vi "test Cancelling an Already Cancelled Test Is A No Op.vi"(8 "error in (no error)":errorcluster, 11 "TestCase in":refnum<class "Cancellation Tests.lvclass">) -> (0 "error out":errorcluster, 3 "TestCase out":refnum<class "Cancellation Tests.lvclass">)   [LabVIEW 2017, in "Cancellation Tests.lvclass"]
uses:
  Cancellation Tests.lvclass
  <vilib>/addons/_JKI Toolkits/VI Tester/TestCase.llb/TestCase.lvclass
  Futures/Futures.lvlib
  Futures/Future/Future.lvclass
  C:/Program Files (x86)/National Instruments/LabVIEW 2017/vi.lib/addons/_JKI Toolkits/VI Tester/TestCase.llb/TestCase.lvclass
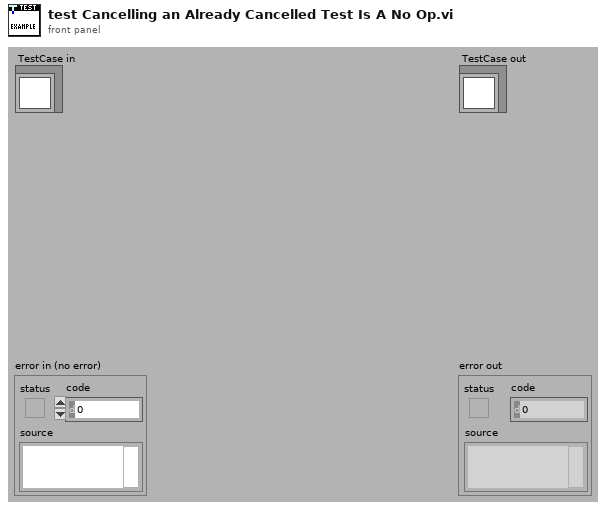
[diagram p1: front panel]
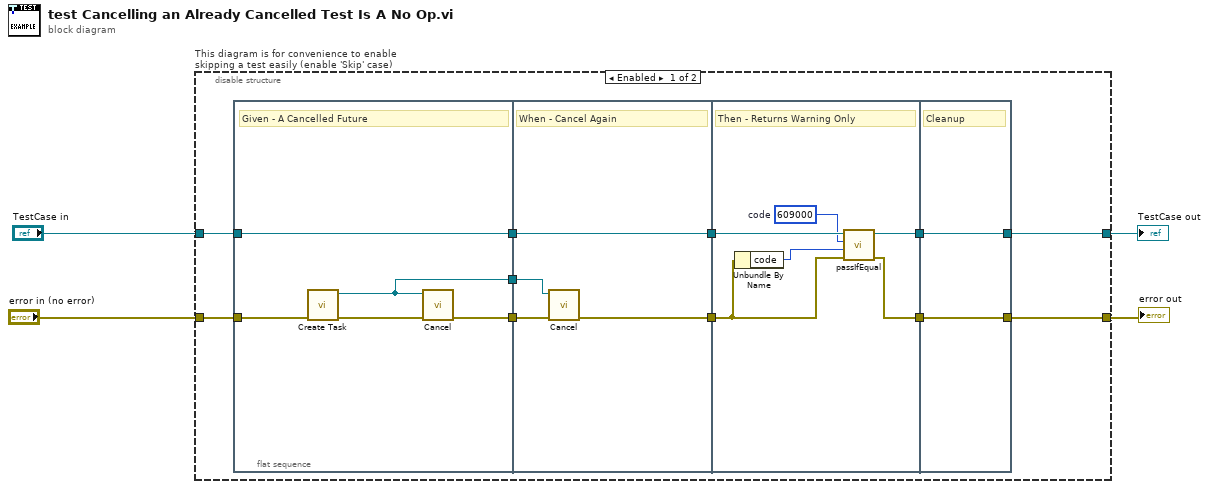
[diagram p0: block diagram]
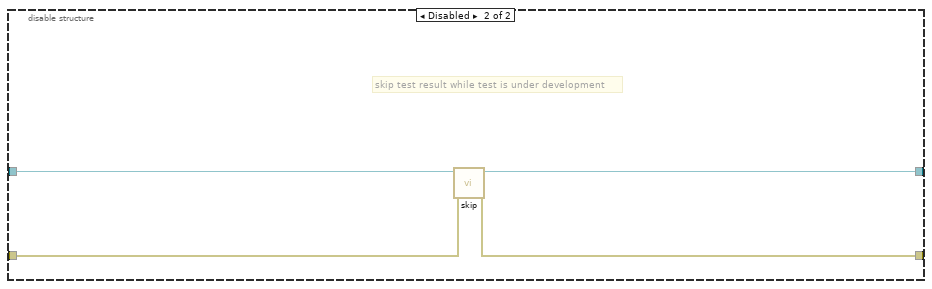
[diagram p2: hidden frame]
diagram:
  n1 = disable-structure "This diagram is for convenience to enable skipping a test easily (enable 'Skip' case)" shown="Enabled" {
    disable-tunnel: "TestCase in" -> [w11 w36]
    disable-tunnel: [w9 w34] -> w1
    disable-tunnel: [w8 w35] -> w3
    disable-tunnel: "error in (no error)" -> [w10 w33]
    frame Enabled {
      n2 = flat-sequence {
        tunnel: w10 -> [w19]
        tunnel: w11 -> [w20]
        tunnel: [w20] -> w15
        tunnel: [w17] -> w7
        tunnel: [w16] -> w6
        tunnel: [w24] -> w14
        tunnel: w15 -> [w24]
        tunnel: w7 -> [w23]
        tunnel: w6 -> [w22]
        tunnel: [w21] -> w5
        tunnel: [w28] -> w13
        tunnel: [w30] -> w12
        tunnel: w14 -> [w29]
        tunnel: w5 -> [w27]
        tunnel: [w31] -> w8
        tunnel: [w32] -> w9
        tunnel: w13 -> [w32]
        tunnel: w12 -> [w31]
        frame #0 {
          # "Given - A Cancelled Future"
          n3 = call "Create Task.vi"("error in (no error)"=w19) -> ("error out"=w18:errorcluster, "Future out"=w16:refnum<class "Future.lvclass">)  [unwired: 8 in, 1 out]
          n4 = call "Cancel.vi"("error in (no error)"=w18, "Future in"=w16) -> ("error out"=w17:errorcluster)  [unwired: 9 in]
        }
        frame #1 {
          # "When - Cancel Again"
          n5 = call "Cancel.vi"("error in (no error)"=w23, "Future in"=w22) -> ("error out"=w21:errorcluster)  [unwired: 9 in]
        }
        frame #2 {
          w25 = 609000  # code
          # "Then - Returns Warning Only"
          n6 = Unbundle By Name(w27) -> ("code"=w26:i32)
          n7 = call-dynamic "passIfEqual.vi"("error in (no error)"=w27, "y"=w26, "x"=w25, "TestCase in"=w29) -> ("error out"=w30:errorcluster, "TestCase out"=w28:refnum<class "Cancellation Tests.lvclass">)  [unwired: 6 in]
        }
        frame #3 {
          # "Cleanup"
        }
      }
    }
    frame Disabled {
      # "skip test result while test is under development"
      n8 = call <vilib>:"skip.vi"("error in (no error)"=w33, "TestCase in"=w36) -> ("error out"=w35:errorcluster, "TestCase out"=w34:refnum<class "Cancellation Tests.lvclass">)  [unwired: 8 in]
    }
  }
  "error out" <- w3
  "TestCase out" <- w1
